vi "connection.vi"(10 "VersionControl":bool, 11 "paramUnicorn in":T1) -> (0 "error out":errorcluster, 3 "paramUnicorn out":T1)   [LabVIEW 2017]
uses:
  Unicorn Labview Library/Control/unicorn_Param.ctl
  Unicorn Labview Library/Control/unicorn_conn.ctl
  Unicorn Labview Library/Control/unicorn_JSON.ctl
  Unicorn Labview Library/Control/unicorn_ParamInt.ctl
  Unicorn Labview Library/Control/unicorn_Telemetry.ctl
  Unicorn Labview Library/Control/unicorn_Table.ctl
  Unicorn Labview Library/Control/unicorn_ParamFloat.ctl
  Unicorn Labview Library/Unicorn Library.lvlib
panel:
  in  "error IO":errorcluster
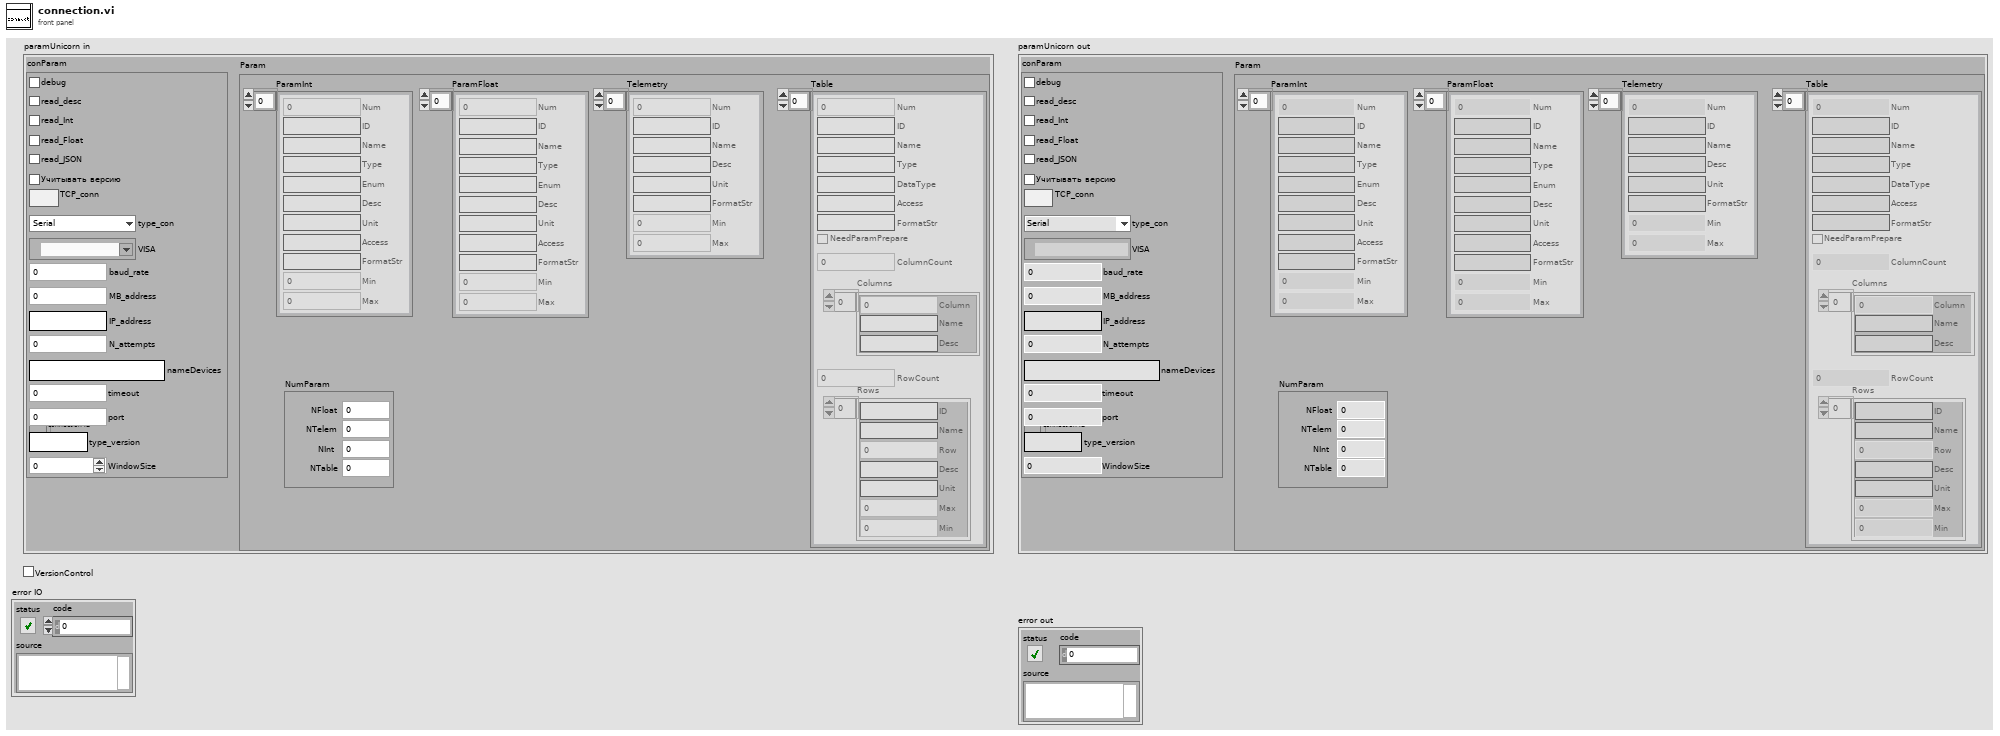
[diagram p1: front panel]
types:
  T1 = typedef "Unicorn Library.lvlib/unicorn_Param.ctl" = cluster{"conParam":T2, "Param":T3}
  T2 = typedef "Unicorn Library.lvlib/unicorn_conn.ctl" = cluster{"ReadIntParam":bool, "ReadDescrParam":bool, "ReadFloatParam":bool, "debug":bool, "ReadJSON":bool, "IP_address":string, "N_attempts":i32, "type_con":enum16{"Serial", "TCP"}, "MB_address":i32, "VISA":refnum<visa-resource-name>, "connection ID":refnum<k5>, "nameDevices":string, "timeout":i32, "port":u16, "type_version":string, "baud_rate":u32, "VersionControl":bool, "TCP_conn":bool, "WindowSize":i32}
  T3 = typedef "Unicorn Library.lvlib/unicorn_JSON.ctl" = cluster{"NumParam":cluster{"NTelem":i32, "NInt":i32, "NFloat":i32, "NTable":i32}, "ParamInt":T4, "Telemetry":T5, "Table":T6, "ParamFloat":T7}
  T4 = typedef "Unicorn Library.lvlib/unicorn_ParamInt.ctl" = cluster{"ID":string, "Num":i32, "Name":string, "Type":string, "Enum":string, "Desc":string, "Unit":string, "Access":string, "FormatStr":string, "Min":i32, "Max":i32}[]
  T5 = typedef "Unicorn Library.lvlib/unicorn_Telemetry.ctl" = cluster{"ID":string, "Num":i32, "Name":string, "Desc":string, "Unit":string, "FormatStr":string, "Min":i32, "Max":i32}[]
  T6 = typedef "Unicorn Library.lvlib/unicorn_Table.ctl" = cluster{"Num":i32, "Access":string, "ColumnCount":i32, "NeedParamPrepare":bool, "Columns":cluster{"Column":i32, "Desc":string, "Name":string}[], "DataType":string, "FormatStr":string, "ID":string, "Name":string, "RowCount":i32, "Rows":cluster{"Desc":string, "ID":string, "Max":i32, "Min":i32, "Name":string, "Row":i32, "Unit":string}[], "Type":string}[]
  T7 = typedef "Unicorn Library.lvlib/unicorn_ParamFloat.ctl" = cluster{"ID":string, "Num":i32, "Name":string, "Type":string, "Enum":string, "Desc":string, "Unit":string, "Access":string, "FormatStr":string, "Min":i32, "Max":i32}[]
  T8 = typedef "Unicorn Library.lvlib/AnswerUDP.ctl" = cluster{"IP":string, "Port":u16, "DataVersion":u16, "ModbusAddress":i32, "type_version":string, "Description":string, "Serial":string, "ServerPort":u16}
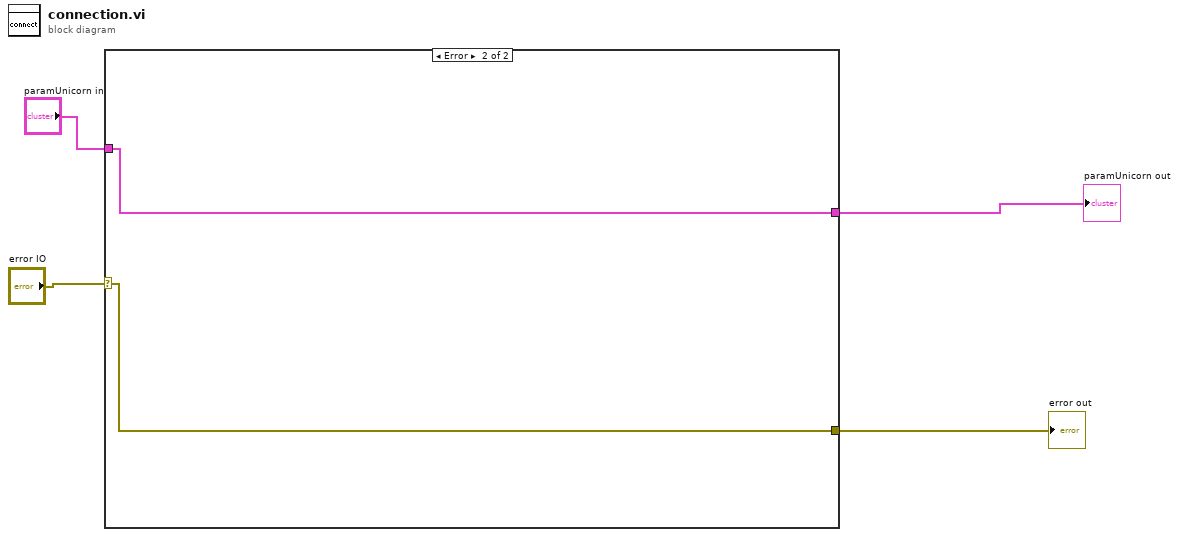
[diagram p0: block diagram]
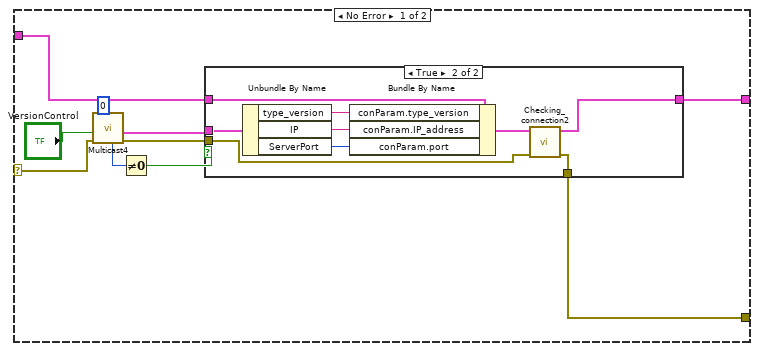
[diagram p2: hidden frame]
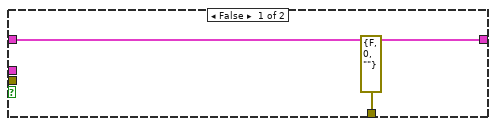
[diagram p3: hidden frame]
diagram:
  n1 = case shown="Error" "error IO" {
    selector: "error IO" -> [w5 w26]
    tunnel: [w14 w26] -> w4
    tunnel: [w12 w27] -> w3
    tunnel: "paramUnicorn in" -> [w8 w27]
    frame No Error {
      n2 = call "Multicast4.vi"("error in"=w5, "VersionControl"="VersionControl", "type_version"=u32 0) -> ("error out"=w13:errorcluster, "selDevice"=w7:T8, "selIPhex"=w9:u32)  [unwired: 3 in, 3 out]
      n3 = Not Equal To 0?(x=w9) -> (x != 0?=w10:bool)
      n4 = case shown="True" w10 {
        tunnel: w7 -> [_ w24]
        tunnel: w8 -> [w16 w23]
        tunnel: [w16 w22] -> w12
        tunnel: w13 -> [_ w18]
        tunnel: [errorcluster {"status"=FALSE, "code"=0, "source"=""} ("error out") w17] -> w14
        frame False {
        }
        frame True {
          n5 = Unbundle By Name(w24) -> ("type_version"=w20:string, "IP"=w21:string, "ServerPort"=w19:u16)
          n6 = Bundle By Name(cluster=w23, "conParam.type_version"=w20, "conParam.IP_address"=w21, "conParam.port"=w19) -> (w25:T1)
          n7 = call "Checking_connection2.vi"("error in"=w18, "paramUnicornIn"=w25) -> ("error out"=w17:errorcluster, "paramUnicorn"=w22:T1)  [unwired: 6 in, 2 out]
        }
      }
    }
    frame Error {
    }
  }
  "error out" <- w4
  "paramUnicorn out" <- w3
